vi "sub_conv_map_gen_v2.vi"(11 "code type":T1(ring)) -> (1 "output in decimal":u32[][](array[numeric]), 3 "state transition":u32[][](array[numeric]))   [LabVIEW 2014]
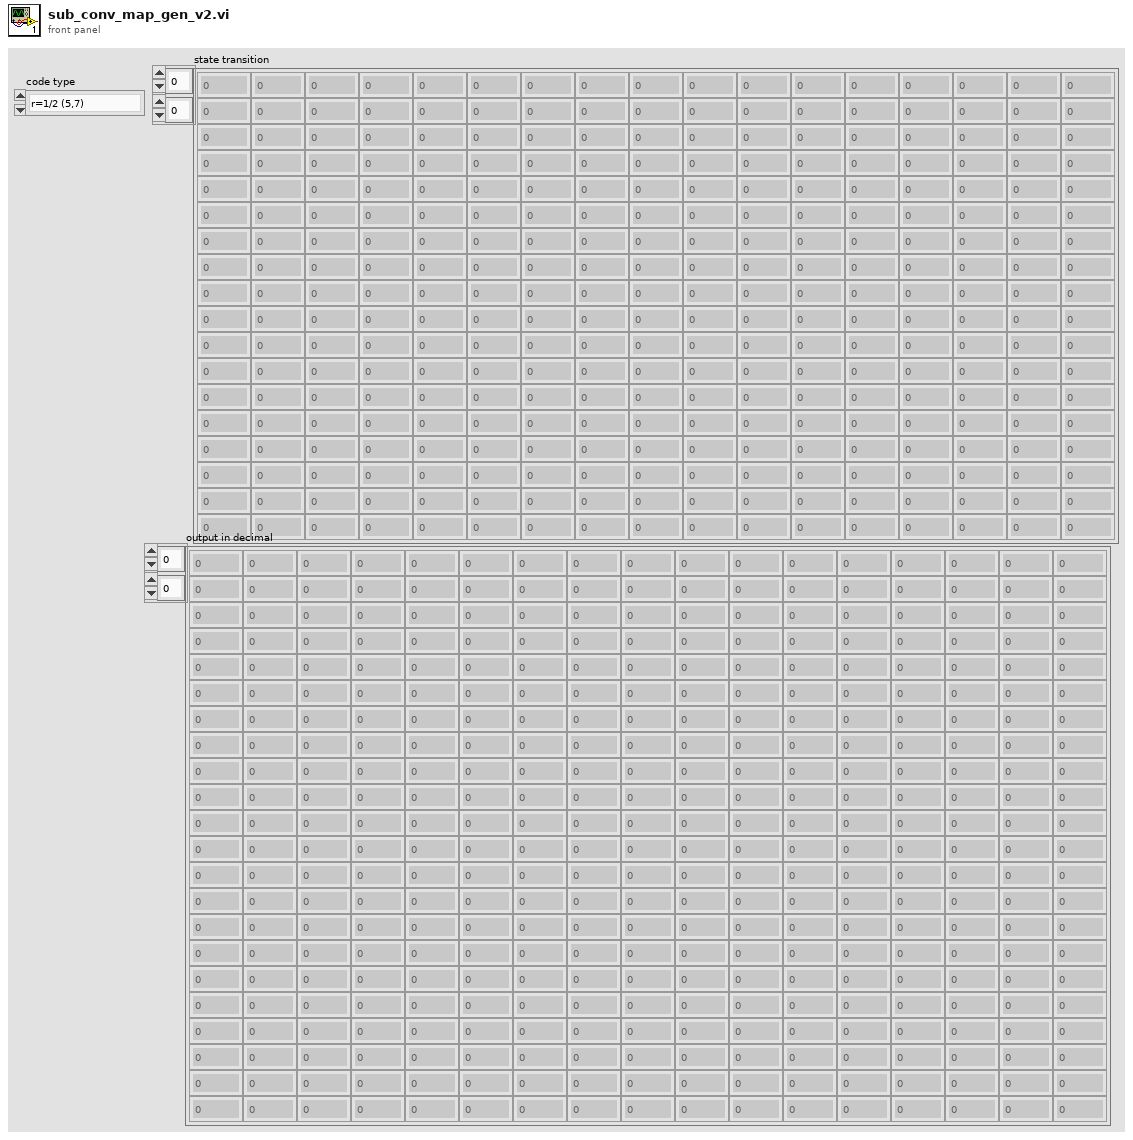
[diagram p1: front panel]
types:
  T1 = enum16{"r=1/2 (5,7)", "r=1/2 (13,17)", "r=1/4 (25,27,33,37)"}
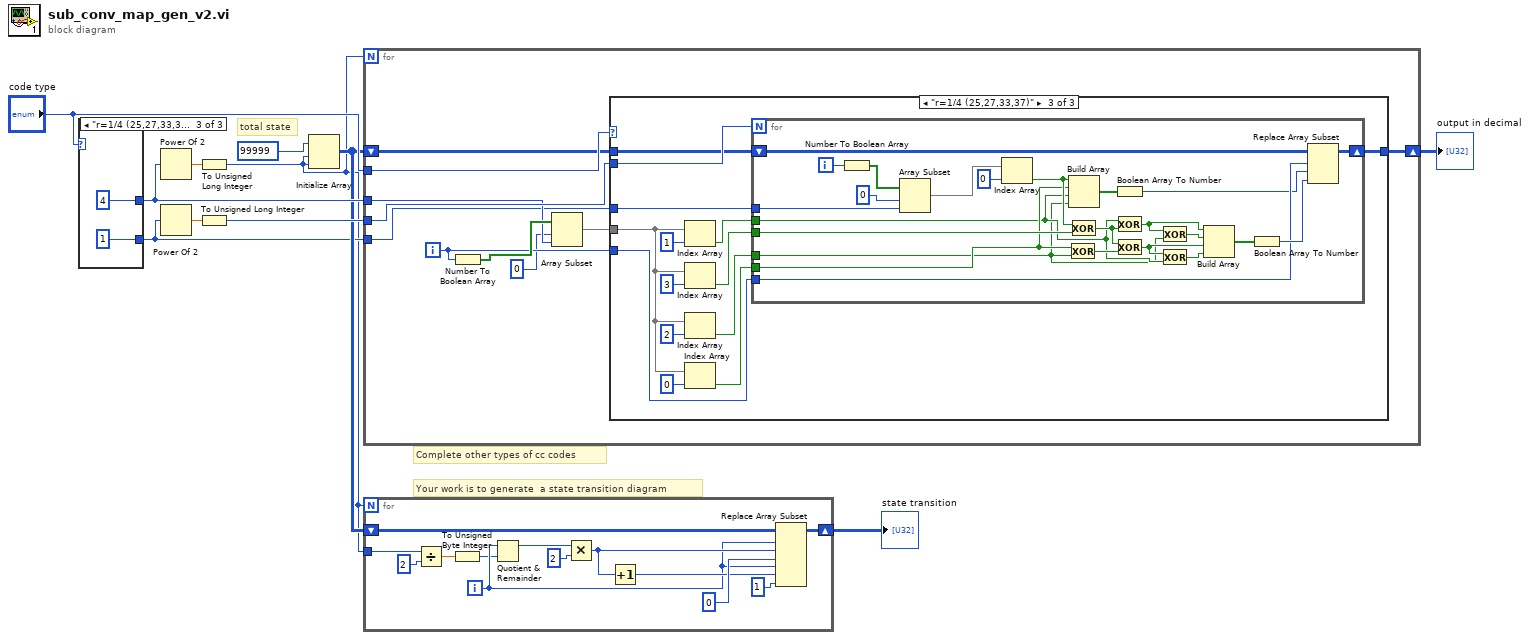
[diagram p0: block diagram]
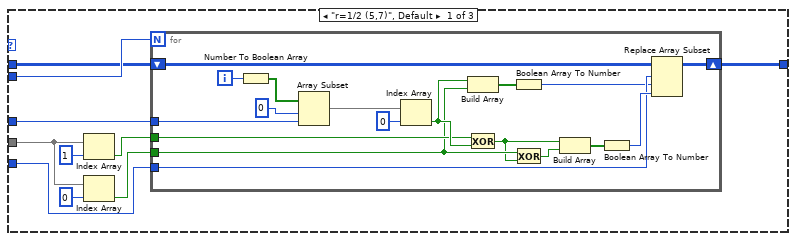
[diagram p2: hidden frame]
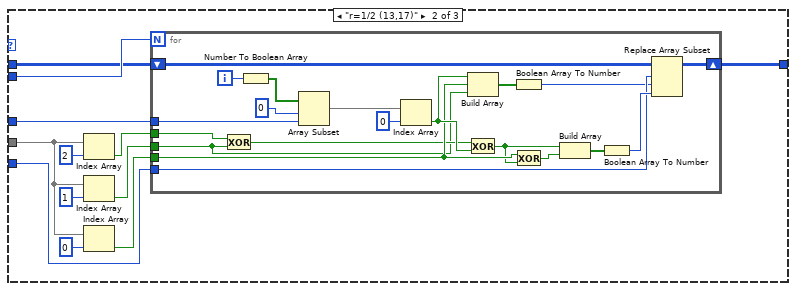
[diagram p3: hidden frame]
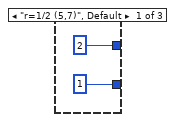
[diagram p4: hidden frame]
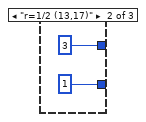
[diagram p5: hidden frame]
diagram:
  # "Your work is to generate  a state transition diagram"
  # "Complete other types of cc codes"
  # "total state"
  n1 = case shown="\"r=1/4 (25,27,33,37)\"" "code type" {
    tunnel: [u32 2 u32 3 u32 4] -> w9
    tunnel: [u32 1 u32 1 u32 1] -> w2
    frame "r=1/2 (5,7)", Default {
    }
    frame "r=1/2 (13,17)" {
    }
    frame "r=1/4 (25,27,33,37)" {
    }
  }
  n2 = Power Of 2(x=w9) -> (2^x=w7:dbl)
  n3 = Power Of 2(x=w2) -> (2^x=w6:dbl)
  n4 = To Unsigned Long Integer(number=w7) -> (unsigned 32bit integer=w1:u32)
  n5 = To Unsigned Long Integer(number=w6) -> (unsigned 32bit integer=w5:u32)
  n6 = Initialize Array(u32 99999, w1, w1) -> (w4:u32[][])
  n7 = for {
    N: w1 -> [_]
    tunnel: w5 -> [w27]
    tunnel: w2 -> [w19]
    tunnel: w9 -> [w25]
    tunnel: "code type" -> [w23]
    shift-right: [w21] -> w3
    shift-left: w4 -> [w22]
    i -> [w20]
    n8 = Number To Boolean Array(number=w20) -> (Boolean array=w26:bool[])
    n9 = Array Subset(array=w26, index=0, length=w25) -> (w24:bool[])
    n10 = case shown="\"r=1/4 (25,27,33,37)\"" w23 {
      tunnel: w27 -> [w37 w63 w95]
      tunnel: w19 -> [w36 w60 w92]
      tunnel: w24 -> [w35 w58 w90]
      tunnel: [w28 w59 w91] -> w21
      tunnel: w22 -> [w30 w62 w94]
      tunnel: w20 -> [w29 w61 w93]
      frame "r=1/2 (5,7)", Default {
        n11 = Index Array(array=w35, index=1) -> (element=w31:bool)
        n12 = Index Array(array=w35, index=0) -> (element=w32:bool)
        n13 = for {
          N: w37 -> [_]
          tunnel: w36 -> [w52]
          tunnel: w31 -> [w41]
          tunnel: w32 -> [w40]
          shift-right: [w43] -> w28
          shift-left: w30 -> [w47]
          tunnel: w29 -> [w45]
          i -> [w55]
          n14 = Number To Boolean Array(number=w55) -> (Boolean array=w54:bool[])
          n15 = Array Subset(array=w54, index=0, length=w52) -> (w51:bool[])
          n16 = Index Array(array=w51, index=0) -> (element=w42:bool)
          n17 = Build Array(w42, w40) -> (w48:bool[])
          n18 = Exclusive Or(1:w42, 2:w41) -> (0:w38:bool)
          n19 = Boolean Array To Number(Boolean array=w48) -> (number=w44:u32)
          n20 = Exclusive Or(1:w38, 2:w40) -> (0:w39:bool)
          n21 = Build Array(w38, w39) -> (w49:bool[])
          n22 = Boolean Array To Number(Boolean array=w49) -> (number=w46:u32)
          n23 = Replace Array Subset(array=w47, new element=w46, index (row)=w45, index (col)=w44) -> (w43:u32[][])
        }
      }
      frame "r=1/2 (13,17)" {
        n24 = Index Array(array=w58, index=2) -> (element=w56:bool)
        n25 = Index Array(array=w58, index=1) -> (element=w64:bool)
        n26 = Index Array(array=w58, index=0) -> (element=w65:bool)
        n27 = for {
          N: w63 -> [_]
          tunnel: w60 -> [w84]
          tunnel: w64 -> [w68]
          tunnel: w65 -> [w73]
          shift-right: [w75] -> w59
          shift-left: w62 -> [w79]
          tunnel: w61 -> [w77]
          tunnel: w56 -> [w70]
          i -> [w87]
          n28 = Exclusive Or(1:w68, 2:w70) -> (0:w69:bool)
          n29 = Number To Boolean Array(number=w87) -> (Boolean array=w86:bool[])
          n30 = Array Subset(array=w86, index=0, length=w84) -> (w83:bool[])
          n31 = Index Array(array=w83, index=0) -> (element=w74:bool)
          n32 = Build Array(w74, w73, w68) -> (w80:bool[])
          n33 = Exclusive Or(1:w74, 2:w69) -> (0:w71:bool)
          n34 = Boolean Array To Number(Boolean array=w80) -> (number=w76:u32)
          n35 = Exclusive Or(1:w71, 2:w73) -> (0:w72:bool)
          n36 = Build Array(w71, w72) -> (w81:bool[])
          n37 = Boolean Array To Number(Boolean array=w81) -> (number=w78:u32)
          n38 = Replace Array Subset(array=w79, new element=w78, index (row)=w77, index (col)=w76) -> (w75:u32[][])
        }
      }
      frame "r=1/4 (25,27,33,37)" {
        n39 = Index Array(array=w90, index=1) -> (element=w98:bool)
        n40 = Index Array(array=w90, index=3) -> (element=w88:bool)
        n41 = Index Array(array=w90, index=2) -> (element=w99:bool)
        n42 = Index Array(array=w90, index=0) -> (element=w96:bool)
        n43 = for {
          N: w95 -> [_]
          tunnel: w92 -> [w122]
          tunnel: w98 -> [w105]
          tunnel: w99 -> [w102]
          shift-right: [w113] -> w91
          shift-left: w94 -> [w117]
          tunnel: w93 -> [w115]
          tunnel: w96 -> [w110]
          tunnel: w88 -> [w111]
          i -> [w125]
          n44 = Number To Boolean Array(number=w125) -> (Boolean array=w124:bool[])
          n45 = Array Subset(array=w124, index=0, length=w122) -> (w121:bool[])
          n46 = Index Array(array=w121, index=0) -> (element=w112:bool)
          n47 = Exclusive Or(1:w102, 2:w110) -> (0:w109:bool)
          n48 = Build Array(w112, w110, w105, w102) -> (w118:bool[])
          n49 = Exclusive Or(1:w111, 2:w112) -> (0:w106:bool)
          n50 = Boolean Array To Number(Boolean array=w118) -> (number=w114:u32)
          n51 = Exclusive Or(1:w106, 2:w105) -> (0:w103:bool)
          n52 = Exclusive Or(1:w109, 2:w106) -> (0:w107:bool)
          n53 = Exclusive Or(1:w102, 2:w103) -> (0:w104:bool)
          n54 = Exclusive Or(1:w105, 2:w107) -> (0:w108:bool)
          n55 = Build Array(w103, w104, w107, w108) -> (w119:bool[])
          n56 = Boolean Array To Number(Boolean array=w119) -> (number=w116:u32)
          n57 = Replace Array Subset(array=w117, new element=w116, index (row)=w115, index (col)=w114) -> (w113:u32[][])
        }
      }
    }
  }
  "output in decimal" <- w3
  n58 = for {
    N: w1 -> [_]
    shift-right: [w131] -> w10
    shift-left: w4 -> [w138]
    tunnel: w1 -> [w130]
    i -> [w132]
    n59 = Divide(x=w130, y=2) -> (x/y=w127:dbl)
    n60 = To Unsigned Byte Integer(number=w127) -> (unsigned 8bit integer=w128:u8)
    n61 = Quotient & Remainder(x=w132, y=w128) -> (x-y*floor(x/y)=w136:i32)  [unwired: 1 out]
    n62 = Multiply(x=w136, y=2) -> (x*y=w135:i32)
    n63 = Increment(x=w135) -> (x+1=w134:i32)
    n64 = Replace Array Subset(array=w138, new element #1=0, index (row) #1=w132, index (col) #1=w135, new element #2=1, index (row) #2=w132, index (col) #2=w134) -> (w131:u32[][])
  }
  "state transition" <- w10
